vi "Ros-Communication.vi"() -> ()   [LabVIEW 2016]
uses:
  <userlib>/ROS for LabVIEW Software/ROS/Code/SubVIs/_ROSControl.ctl
  <userlib>/ROS for LabVIEW Software/ROS/Code/SubVIs/_ROSDirection.ctl
  <userlib>/ROS for LabVIEW Software/ROS/Code/Console/Servers/ServerSubs/TopicDef.ctl
panel:
  in  "stop":bool
  out "ROS out":T1={"topic port"=0, "Node"="", "topic"="", "type"="", "node port"=0, "error "={"status"=FALSE, "code"=0, "source"=""}, "Direction"=enum."Node", "Update (ms)"=1, "FIFO size"=1}
  in  "Twist":T3
  out "error out":errorcluster
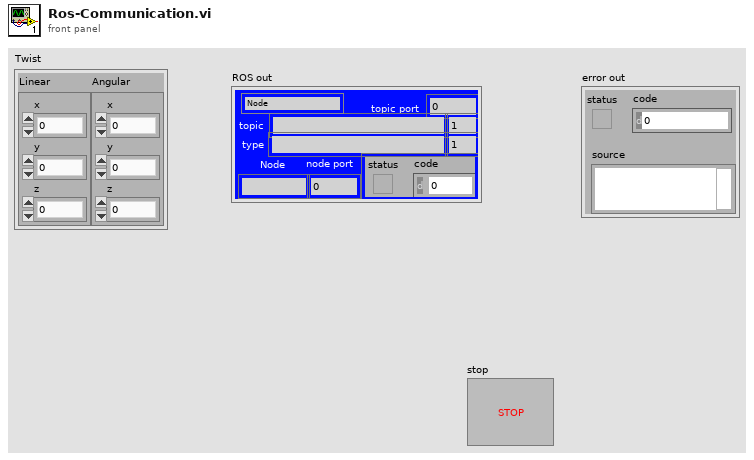
[diagram p1: front panel]
types:
  T1 = typedef "_ROSControl.ctl" = cluster{"topic port":u16, "Node":string, "topic":string, "type":string, "node port":u16, "error ":errorcluster, "Direction":T2, "Update (ms)":u16, "FIFO size":u16}
  T2 = typedef "_ROSDirection.ctl" = enum16{"Node", "Publisher", "Subscriber", "ServiceClient", "ServiceProvider"}
  T3 = cluster{"Linear":cluster{"x":dbl, "y":dbl, "z":dbl}, "Angular":cluster{"x":dbl, "y":dbl, "z":dbl}}
  T4 = typedef "TopicDef.ctl" = cluster{"Topic":string, "Type":string, "Action":T2, "Update (ms)":u16, "queue size":u16}
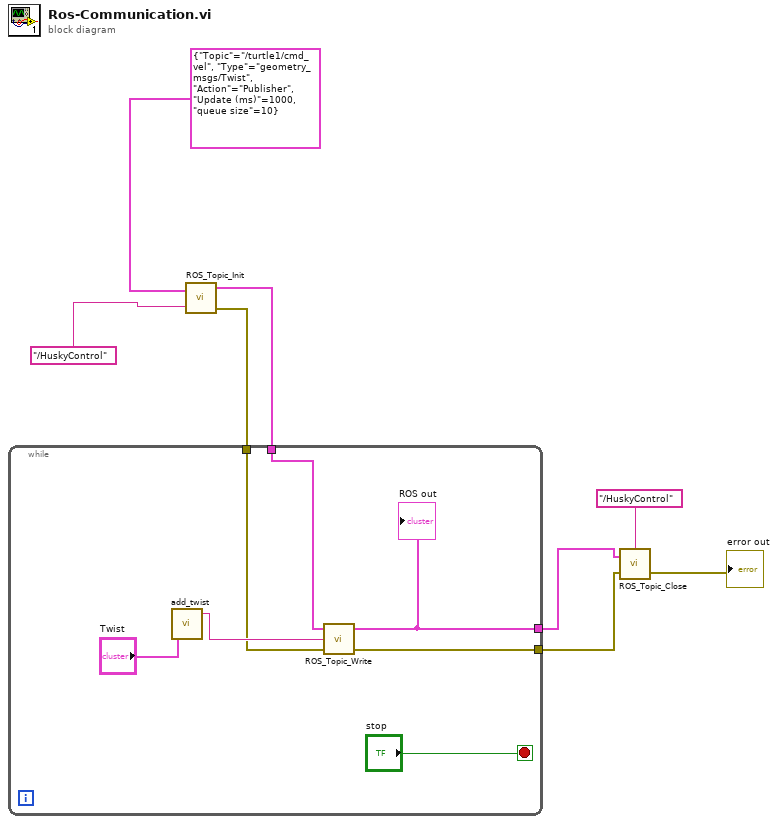
[diagram p0: block diagram]
diagram:
  n1 = call <userlib>:"ROS_Topic_Init.vi"("Definitions"=T4 {"Topic"="/turtle1/cmd_vel", "Type"="geometry_msgs/Twist", "Action"=enum."Publisher", "Update (ms)"=1000, "queue size"=10}, "node"="/HuskyControl") -> ("ROS out"=w5:T1, "error out"=w4:errorcluster)  [unwired: 1 in]
  n2 = while {
    tunnel: w5 -> [w12]
    tunnel: w4 -> [w13]
    tunnel: [w11] -> w2
    tunnel: [w10] -> w1
    stop <- "stop" stop-if-true
    n3 = call <userlib>:"add_twist.vi"("Twist"="Twist") -> ("msg out"=w14:string)  [unwired: 4 in]
    n4 = call <userlib>:"ROS_Topic_Write.vi"("error in (no error)"=w13, "Msg in"=w14, "ROS in"=w12) -> ("error out"=w10:errorcluster, "ROS out"=w11:T1)  [unwired: 1 in]
    "ROS out" <- w11
  }
  n5 = call <userlib>:"ROS_Topic_Close.vi"("error in"=w1, "ROS in"=w2, "node"="/HuskyControl") -> ("error out"=→"error out":errorcluster)  [unwired: 1 in]
